vi "Periodic Tasks.vi"(8 "error in":errorcluster) -> ()   [LabVIEW 2019]
doc: "This VI runs in parallel to other tasks. It can contain as many user-defined periodic loops as you need. These can carry out PID or other sorts of timed response."
uses:
  <vilib>/Rock Robotics/WPI/Utilities/WPI_GetSetVariantRefNum.vi
  <vilib>/Rock Robotics/WPI/ThirdParty/Phoenix-LabVIEW/Motor Controller/Controls/CTRE_Phoenix_MotorControl_ControlMode.ctl
  <vilib>/Rock Robotics/WPI/ThirdParty/Phoenix-LabVIEW/Motor Controller/Controls/CTRE_Phoenix_MotorControl_RemoteFeedbackDevice.ctl
  <vilib>/Rock Robotics/WPI/ThirdParty/Phoenix-LabVIEW/Motor Controller/Controls/CTRE_Phoenix_MotorControl_RemoteSourceType.ctl
  <vilib>/Rock Robotics/WPI/ThirdParty/Phoenix-LabVIEW/Controls/CTRE_Phoenix_Params.ctl
panel:
  in  "Forward Limit Threshold":i32
  in  "Reverse Limit Threshold":i32
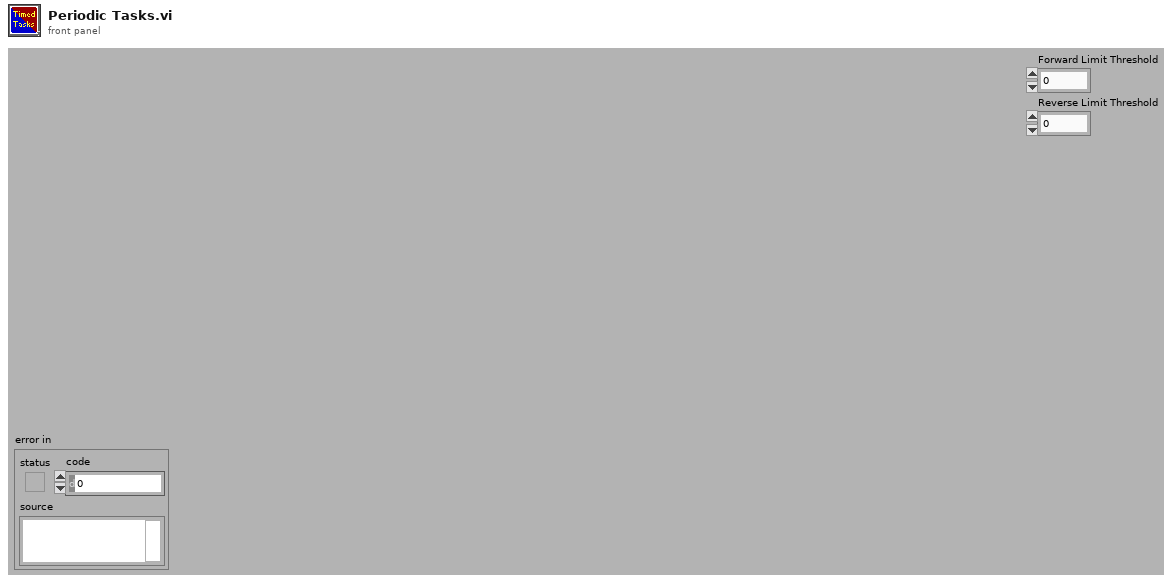
[diagram p1: front panel]
types:
  T1 = typedef "CTRE_PigeonIMU_DeviceRef.ctl" = cluster{"DeviceStatus":errorcluster, "Device Number":u8, "Type":T2, "Device ID":u32, "Handle":u64, "UsageFrame":u32, "Library Path":path}
  T2 = typedef "CTRE_PigeonIMU_ConnectionType.ctl" = u32
  T3 = typedef "CTRE_CANifier_DeviceRef.ctl" = cluster{"DeviceStatus":errorcluster, "Device Number":u8, "Handle":u64, "UsageFrame":u32, "Library Path":path}
  T4 = typedef "WPI_MotorControlDeviceRef.ctl" = cluster{"DeviceStatus":errorcluster, "Type":T5, "PWM":cluster{"PWM Channel":T6, "DeadBand":T7}, "CAN":cluster{"Device Number":u8, "SetOutput VI Ref":variant, "GetOutput VI Ref":variant, "Enable VI Ref":variant, "Disable VI Ref":variant, "Data":variant}, "Invert":bool, "DIO PWM":cluster{"PWM \"Enable\" Channel":T6, "DIOChannel":T8, "PWM Rate":dbl}}
  T5 = typedef "WPI_MotorControlType.ctl" = enum16{"PWM", "CAN", "DIO PWM"}
  T6 = typedef "FPGA_DIOPWMChannel.ctl" = enum8{"PWM 0", "PWM 1", "PWM 2", "PWM 3", "PWM 4", "PWM 5", "PWM 6", "PWM 7", "PWM 8", "PWM 9", "PWM MXP 0", "PWM MXP 1", "PWM MXP 2", "PWM MXP 3", "PWM MXP 4", "PWM MXP 5", "PWM MXP 6", "PWM MXP 7", "PWM MXP 8", "PWM MXP 9", "Invalid"}
  T7 = typedef "WPI_PWMDeadband.ctl" = cluster{"Name":string, "maxPositivePwm":i32, "minPositivePwm":i32, "centerPwm":i32, "maxNegativePwm":i32, "minNegativePwm":i32, "angularRange":u16}
  T8 = typedef "FPGA_DIOChannel.ctl" = enum8{"DIO 0", "DIO 1", "DIO 2", "DIO 3", "DIO 4", "DIO 5", "DIO 6", "DIO 7", "DIO 8", "DIO 9", "DIO MXP 0", "DIO MXP 1", "DIO MXP 2", "DIO MXP 3", "DIO MXP 4", "DIO MXP 5", "DIO MXP 6", "DIO MXP 7", "DIO MXP 8", "DIO MXP 9", "DIO MXP 10", "DIO MXP 11", "DIO MXP 12", "DIO MXP 13", "DIO MXP 14", "DIO MXP 15", "SPI Port CS1", "SPI Port CS2", "SPI Port CS3", "SPI Port MISO", "SPI Port MOSI", "Invalid"}
  T9 = typedef "WPI_JoystickDevRef.ctl" = cluster{"Device":T10}
  T10 = typedef "WPI_JoystickDeviceEnum.ctl" = enum16{"USB 0", "USB 1", "USB 2", "USB 3", "USB 4", "USB 5"}
  T11 = typedef "CTRE_Phoenix_MotorControl_RemoteSourceType.ctl" = enum16{"Off", "Talon SRX Selected Sensor", "Pigeon IMU Yaw", "Pigeon IMU Pitch", "Pigeon IMU Roll", "CANifier Quadrature", "CANifier PWM Input 0", "CANifier PWM Input 1", "CANifier PWM Input 2", "CANifier PWM Input 3", "Gadgeteer Pigeon Yaw", "Gadgeteer Pigeon Pitch", "Gadgeteer Pigeon Roll"}
  T12 = typedef "CTRE_Phoenix_MotorControl_ControlMode.ctl" = u16
  T13 = typedef "CTRE_Phoenix_MotorControl_RemoteFeedbackDevice.ctl" = i8
  T14 = typedef "CTRE_Phoenix_Params.ctl" = u16
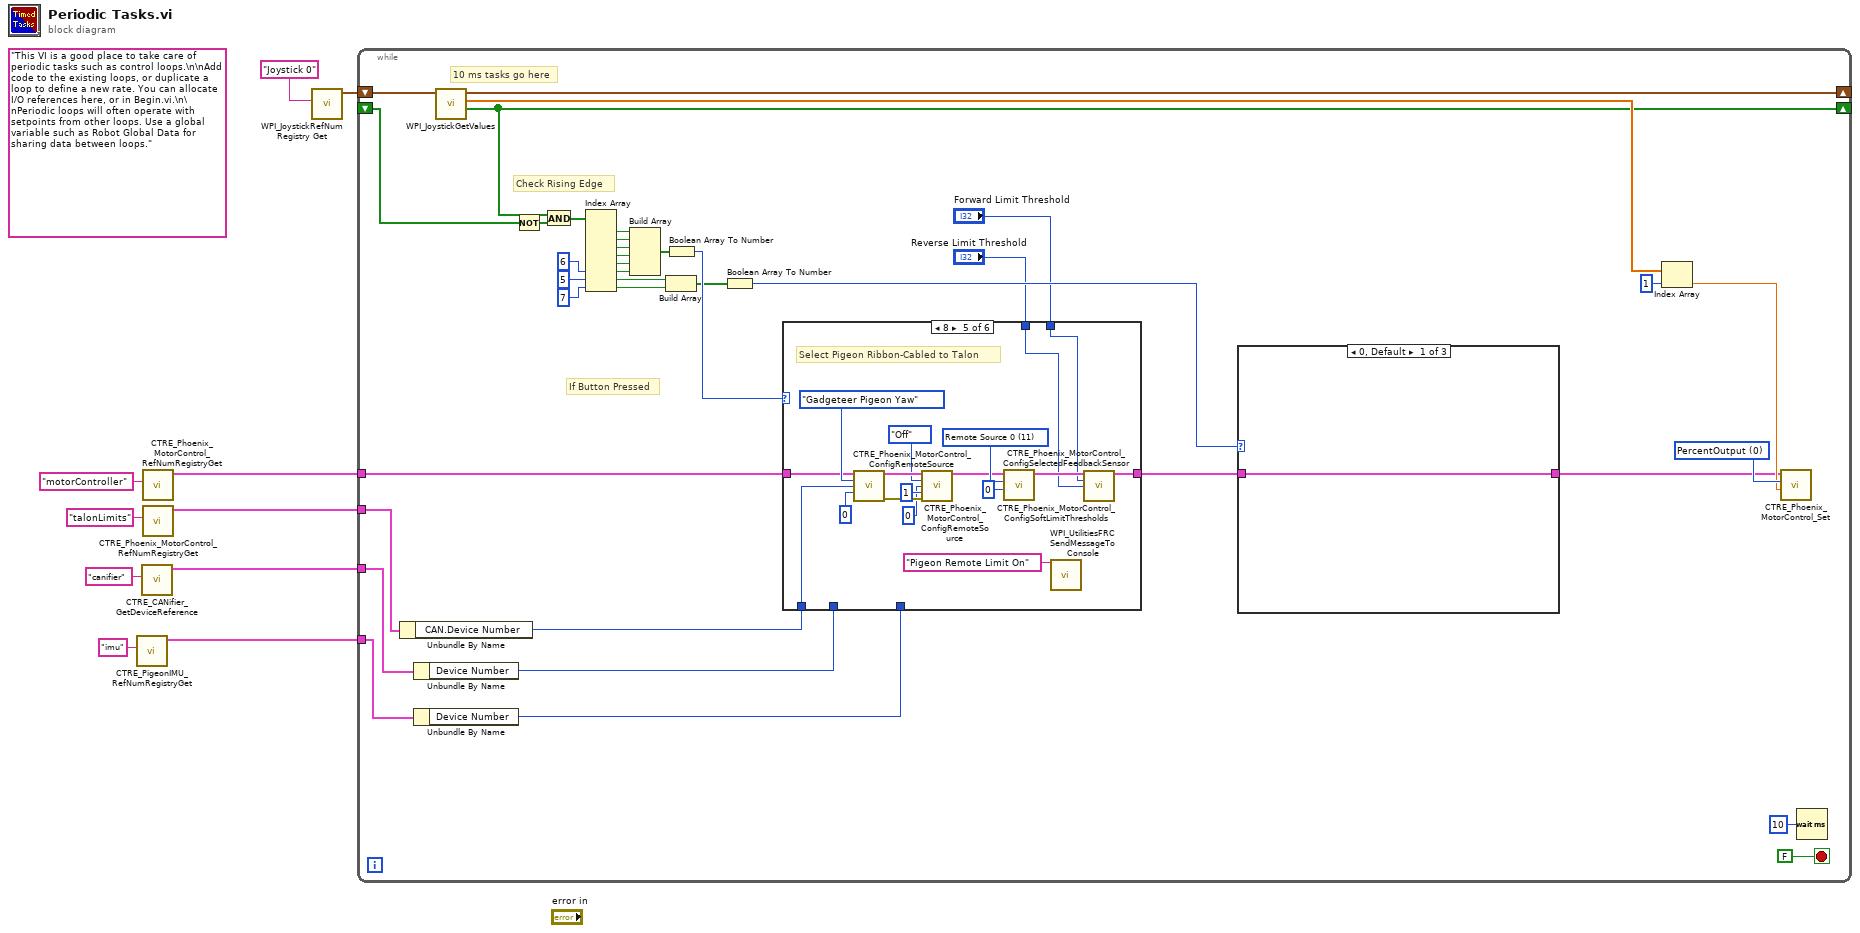
[diagram p0: block diagram]
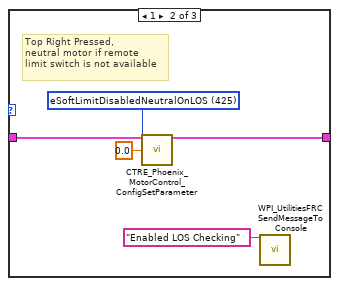
[diagram p2: hidden frame]
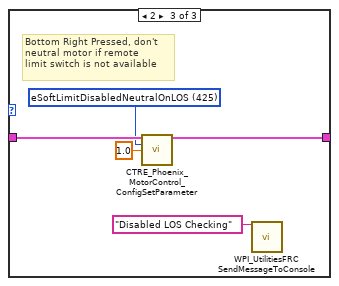
[diagram p3: hidden frame]
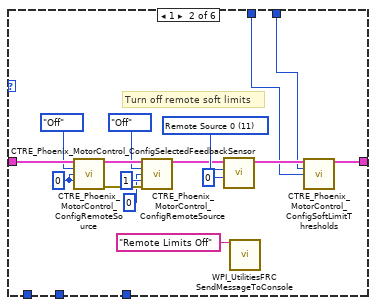
[diagram p5: hidden frame]
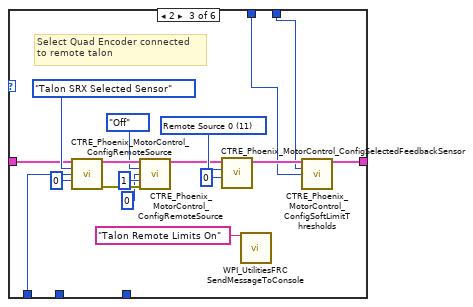
[diagram p6: hidden frame]
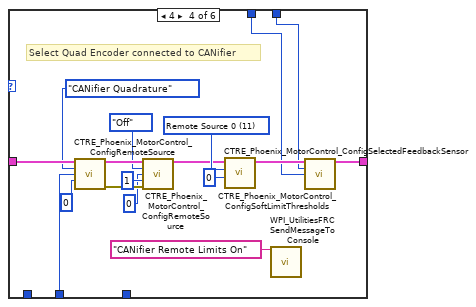
[diagram p7: hidden frame]
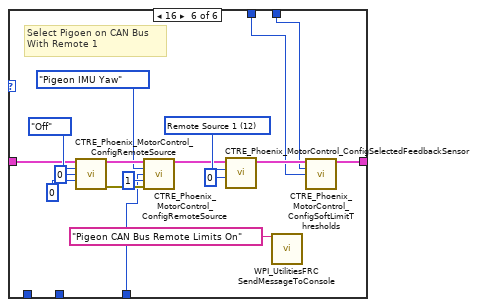
[diagram p8: hidden frame]
diagram:
  (unwired) "This VI is a good place to take care of periodic tasks such as control loops.\n\nAdd code to the existing loops, or duplicate a loop to define a new rate. You can allocate I/O references here, or in Begin.vi.\n\nPeriodic loops will often operate with setpoints from other loops. Use a global variable such as Robot Global Data for sharing data between loops."
  n1 = call <vilib>:"CTRE_PigeonIMU_RefNumRegistryGet.vi"("refnum name"="imu") -> ("PigeonIMUDevRef"=w1:T1)  [unwired: 9 in, 1 out]
  n2 = call <vilib>:"CTRE_CANifier_GetDeviceReference.vi"("refnum name"="canifier") -> ("CANifierDevRef"=w5:T3)  [unwired: 9 in, 1 out]
  n3 = call <vilib>:"CTRE_Phoenix_MotorControl_RefNumRegistryGet.vi"("refnum name"="motorController") -> ("PhoenixMotorControlDevRef"=w3:T4)  [unwired: 9 in, 1 out]
  n4 = call <vilib>:"CTRE_Phoenix_MotorControl_RefNumRegistryGet.vi"("refnum name"="talonLimits") -> ("PhoenixMotorControlDevRef"=w4:T4)  [unwired: 9 in, 1 out]
  n5 = call <vilib>:"WPI_JoystickRefNum Registry Get.vi"("refnum name"="Joystick 0") -> ("JoystickDevRef"=w9:T9)  [unwired: 1 in, 9 out]
  n6 = while {
    shift-right: [w44] -> _
    shift-left: w9 -> [w45]
    tunnel: w5 -> [w34]
    tunnel: w4 -> [w35]
    tunnel: w3 -> [w36]
    shift-right: [w39] -> _
    shift-left: _ -> [w40]
    tunnel: w1 -> [w12]
    stop <- FALSE stop-if-true
    w46 = T12 0 items=["PercentOutput"=0, "Position"=1, "Velocity"=2, "Current"=3, "Follower"=5, "MotionProfile"=6, "MotionMagic"=7, "MotionMagicArc"=8, "MotionProfileArc"=10, "Disabled"=15] ("Control Mode")
    # "If Button Pressed"
    # "Check Rising Edge"
    # "10 ms tasks go here"
    n7 = Unbundle By Name(w35) -> ("CAN.Device Number"=w27:u8)
    n8 = Unbundle By Name(w34) -> ("Device Number"=w26:u8)
    n9 = Unbundle By Name(w12) -> ("Device Number"=w11:u8)
    n10 = call <vilib>:"WPI_JoystickGetValues.vi"("JoystickDevRef"=w45) -> ("Buttons"=w39:bool[], "Axes"=w43:dbl[], "JoystickDevRef"=w44:T9)  [unwired: 6 in, 2 out]
    n11 = Not(x=w40) -> (.not. x?=w38:bool[])
    n12 = And(x=w39, y=w38) -> (x .and. y?=w37:bool[])
    n13 = Index Array(array=w37, index #6=6 ("index"), index #7=5 ("index"), index #8=7 ("index")) -> (element #1=w33:bool, element #2=w30:bool, element #3=w31:bool, element #4=w32:bool, element #5=w21:bool, element #6=w20:bool, element #7=w19:bool, element #8=w18:bool)  [unwired: 5 in]
    n14 = Build Array(w33, w30, w31, w32, w21, w20) -> (w29:bool[])
    n15 = Build Array(w19, w18) -> (w25:bool[])
    n16 = Boolean Array To Number(Boolean array=w29) -> (number=w28:u32)
    n17 = Boolean Array To Number(Boolean array=w25) -> (number=w23:u32)
    n18 = case shown="8" w28 {
      tunnel: w36 -> [w60 w75 w80 w100 w117 w134]
      tunnel: w27 -> [_ _ w84 _ w114 _]
      tunnel: w26 -> [_ _ _ w96 _ _]
      tunnel: [w60 w66 w79 w101 w118 w135] -> w22
      tunnel: "Reverse Limit Threshold" -> [_ w64 w82 w97 w116 w131]
      tunnel: "Forward Limit Threshold" -> [_ w65 w83 w98 w115 w132]
      tunnel: w11 -> [_ _ _ _ _ w133]
      frame 0, Default {
        # "Nothing pressed"
      }
      frame 1 {
        w62 = u32 0 ("Source Index (0/1)")
        w76 = T13 11 items=["None"=-1, "Sensor Sum (S0 + S1)"=9, "Sensor Difference (D0 - D1)"=10, "Remote Source 0"=11, "Remote Source 1"=12, "Software Emulated"=15] ("Feedback Device")
        # "Turn off remote soft limits"
        n19 = call <vilib>:"CTRE_Phoenix_MotorControl_ConfigRemoteSource.vi"("PhoenixMotorControlDevRef"=w75, "Remote Device Type"=CTRE_Phoenix_MotorControl_RemoteSourceType."Off", "Remote Device ID"=w62, "Source Index (0/1)"=w62) -> ("PhoenixMotorControlDevRef"=w72:T4, "error out"=w71:errorcluster)  [unwired: 10 in]
        n20 = call <vilib>:"CTRE_Phoenix_MotorControl_ConfigRemoteSource.vi"("PhoenixMotorControlDevRef"=w72, "Remote Device Type"=CTRE_Phoenix_MotorControl_RemoteSourceType."Off", "Remote Device ID"=u8 0, "Source Index (0/1)"=u32 1, "error in (no error)"=w71) -> ("PhoenixMotorControlDevRef"=w69:T4)  [unwired: 9 in, 1 out]
        n21 = call <vilib>:"CTRE_Phoenix_MotorControl_ConfigSelectedFeedbackSensor.vi"("pidLoopIdx"=0, "Feedback Device"=w76, "PhoenixMotorControlDevRef"=w69) -> ("PhoenixMotorControlDevRef"=w67:T4)  [unwired: 7 in, 1 out]
        n22 = call <vilib>:"WPI_UtilitiesFRC SendMessageToConsole.vi"("Message"="Remote Limits Off") -> ()  [unwired: 14 in, 1 out]
        n23 = call <vilib>:"CTRE_Phoenix_MotorControl_ConfigSoftLimitThresholds.vi"("PhoenixMotorControlDevRef"=w67, "Forward Soft Limit"=w65, "Reverse Soft Limit"=w64) -> ("PhoenixMotorControlDevRef"=w66:T4)  [unwired: 11 in, 1 out]
      }
      frame 2 {
        w93 = T13 11 items=["None"=-1, "Sensor Sum (S0 + S1)"=9, "Sensor Difference (D0 - D1)"=10, "Remote Source 0"=11, "Remote Source 1"=12, "Software Emulated"=15] ("Feedback Device")
        # "Select Quad Encoder connected\nto remote talon"
        n24 = call <vilib>:"CTRE_Phoenix_MotorControl_ConfigRemoteSource.vi"("PhoenixMotorControlDevRef"=w80, "Remote Device Type"=CTRE_Phoenix_MotorControl_RemoteSourceType."Talon SRX Selected Sensor", "Remote Device ID"=w84, "Source Index (0/1)"=u32 0) -> ("PhoenixMotorControlDevRef"=w90:T4, "error out"=w89:errorcluster)  [unwired: 10 in]
        n25 = call <vilib>:"CTRE_Phoenix_MotorControl_ConfigRemoteSource.vi"("PhoenixMotorControlDevRef"=w90, "Remote Device Type"=CTRE_Phoenix_MotorControl_RemoteSourceType."Off", "Remote Device ID"=u8 0, "Source Index (0/1)"=u32 1, "error in (no error)"=w89) -> ("PhoenixMotorControlDevRef"=w87:T4)  [unwired: 9 in, 1 out]
        n26 = call <vilib>:"CTRE_Phoenix_MotorControl_ConfigSelectedFeedbackSensor.vi"("pidLoopIdx"=0, "Feedback Device"=w93, "PhoenixMotorControlDevRef"=w87) -> ("PhoenixMotorControlDevRef"=w85:T4)  [unwired: 7 in, 1 out]
        n27 = call <vilib>:"WPI_UtilitiesFRC SendMessageToConsole.vi"("Message"="Talon Remote Limits On") -> ()  [unwired: 14 in, 1 out]
        n28 = call <vilib>:"CTRE_Phoenix_MotorControl_ConfigSoftLimitThresholds.vi"("PhoenixMotorControlDevRef"=w85, "Forward Soft Limit"=w83, "Reverse Soft Limit"=w82) -> ("PhoenixMotorControlDevRef"=w79:T4)  [unwired: 11 in, 1 out]
      }
      frame 4 {
        w110 = T13 11 items=["None"=-1, "Sensor Sum (S0 + S1)"=9, "Sensor Difference (D0 - D1)"=10, "Remote Source 0"=11, "Remote Source 1"=12, "Software Emulated"=15] ("Feedback Device")
        # "Select Quad Encoder connected to CANifier"
        n29 = call <vilib>:"CTRE_Phoenix_MotorControl_ConfigRemoteSource.vi"("PhoenixMotorControlDevRef"=w100, "Remote Device Type"=CTRE_Phoenix_MotorControl_RemoteSourceType."CANifier Quadrature", "Remote Device ID"=w96, "Source Index (0/1)"=u32 0) -> ("PhoenixMotorControlDevRef"=w108:T4, "error out"=w107:errorcluster)  [unwired: 10 in]
        n30 = call <vilib>:"CTRE_Phoenix_MotorControl_ConfigRemoteSource.vi"("PhoenixMotorControlDevRef"=w108, "Remote Device Type"=CTRE_Phoenix_MotorControl_RemoteSourceType."Off", "Remote Device ID"=u8 0, "Source Index (0/1)"=u32 1, "error in (no error)"=w107) -> ("PhoenixMotorControlDevRef"=w105:T4)  [unwired: 9 in, 1 out]
        n31 = call <vilib>:"CTRE_Phoenix_MotorControl_ConfigSelectedFeedbackSensor.vi"("pidLoopIdx"=0, "Feedback Device"=w110, "PhoenixMotorControlDevRef"=w105) -> ("PhoenixMotorControlDevRef"=w103:T4)  [unwired: 7 in, 1 out]
        n32 = call <vilib>:"WPI_UtilitiesFRC SendMessageToConsole.vi"("Message"="CANifier Remote Limits On") -> ()  [unwired: 14 in, 1 out]
        n33 = call <vilib>:"CTRE_Phoenix_MotorControl_ConfigSoftLimitThresholds.vi"("PhoenixMotorControlDevRef"=w103, "Forward Soft Limit"=w98, "Reverse Soft Limit"=w97) -> ("PhoenixMotorControlDevRef"=w101:T4)  [unwired: 11 in, 1 out]
      }
      frame 8 {
        w127 = T13 11 items=["None"=-1, "Sensor Sum (S0 + S1)"=9, "Sensor Difference (D0 - D1)"=10, "Remote Source 0"=11, "Remote Source 1"=12, "Software Emulated"=15] ("Feedback Device")
        # "Select Pigeon Ribbon-Cabled to Talon"
        n34 = call <vilib>:"CTRE_Phoenix_MotorControl_ConfigRemoteSource.vi"("PhoenixMotorControlDevRef"=w117, "Remote Device Type"=CTRE_Phoenix_MotorControl_RemoteSourceType."Gadgeteer Pigeon Yaw", "Remote Device ID"=w114, "Source Index (0/1)"=u32 0) -> ("PhoenixMotorControlDevRef"=w125:T4, "error out"=w124:errorcluster)  [unwired: 10 in]
        n35 = call <vilib>:"CTRE_Phoenix_MotorControl_ConfigRemoteSource.vi"("PhoenixMotorControlDevRef"=w125, "Remote Device Type"=CTRE_Phoenix_MotorControl_RemoteSourceType."Off", "Remote Device ID"=u8 0, "Source Index (0/1)"=u32 1, "error in (no error)"=w124) -> ("PhoenixMotorControlDevRef"=w122:T4)  [unwired: 9 in, 1 out]
        n36 = call <vilib>:"CTRE_Phoenix_MotorControl_ConfigSelectedFeedbackSensor.vi"("pidLoopIdx"=0, "Feedback Device"=w127, "PhoenixMotorControlDevRef"=w122) -> ("PhoenixMotorControlDevRef"=w120:T4)  [unwired: 7 in, 1 out]
        n37 = call <vilib>:"WPI_UtilitiesFRC SendMessageToConsole.vi"("Message"="Pigeon Remote Limit On") -> ()  [unwired: 14 in, 1 out]
        n38 = call <vilib>:"CTRE_Phoenix_MotorControl_ConfigSoftLimitThresholds.vi"("PhoenixMotorControlDevRef"=w120, "Forward Soft Limit"=w115, "Reverse Soft Limit"=w116) -> ("PhoenixMotorControlDevRef"=w118:T4)  [unwired: 11 in, 1 out]
      }
      frame 16 {
        w144 = T13 12 items=["None"=-1, "Sensor Sum (S0 + S1)"=9, "Sensor Difference (D0 - D1)"=10, "Remote Source 0"=11, "Remote Source 1"=12, "Software Emulated"=15] ("Feedback Device")
        # "Select Pigoen on CAN Bus\nWith Remote 1"
        n39 = call <vilib>:"CTRE_Phoenix_MotorControl_ConfigRemoteSource.vi"("PhoenixMotorControlDevRef"=w134, "Remote Device Type"=CTRE_Phoenix_MotorControl_RemoteSourceType."Off", "Remote Device ID"=u8 0, "Source Index (0/1)"=u32 0) -> ("PhoenixMotorControlDevRef"=w142:T4, "error out"=w141:errorcluster)  [unwired: 10 in]
        n40 = call <vilib>:"CTRE_Phoenix_MotorControl_ConfigRemoteSource.vi"("PhoenixMotorControlDevRef"=w142, "Remote Device Type"=CTRE_Phoenix_MotorControl_RemoteSourceType."Pigeon IMU Yaw", "Remote Device ID"=w133, "Source Index (0/1)"=u32 1, "error in (no error)"=w141) -> ("PhoenixMotorControlDevRef"=w139:T4)  [unwired: 9 in, 1 out]
        n41 = call <vilib>:"CTRE_Phoenix_MotorControl_ConfigSelectedFeedbackSensor.vi"("pidLoopIdx"=0, "Feedback Device"=w144, "PhoenixMotorControlDevRef"=w139) -> ("PhoenixMotorControlDevRef"=w137:T4)  [unwired: 7 in, 1 out]
        n42 = call <vilib>:"WPI_UtilitiesFRC SendMessageToConsole.vi"("Message"="Pigeon CAN Bus Remote Limits On") -> ()  [unwired: 14 in, 1 out]
        n43 = call <vilib>:"CTRE_Phoenix_MotorControl_ConfigSoftLimitThresholds.vi"("PhoenixMotorControlDevRef"=w137, "Forward Soft Limit"=w132, "Reverse Soft Limit"=w131) -> ("PhoenixMotorControlDevRef"=w135:T4)  [unwired: 11 in, 1 out]
      }
    }
    n44 = case shown="0, Default" w23 {
      tunnel: [w49 w52 w57] -> w24
      tunnel: w22 -> [w49 w54 w59]
      frame 0, Default {
      }
      frame 1 {
        w51 = T14 425 items=["eOnBoot_BrakeMode"=31, "eQuadFilterEn"=91, "eQuadIdxPolarity"=108, "eClearPositionOnIdx"=100, "eMotionProfileHasUnderrunErr"=119, "eMotionProfileTrajectoryPointDurationMs"=120, "eClearPosOnLimitF"=144, "eClearPosOnLimitR"=145, "eStatusFramePeriod"=300, "eOpenLoopRamp"=301, "eClosedLoopRamp"=302, "eNeutralDeadband"=303, "ePeakPosOutput"=305, "eNominalPosOutput"=306, "ePeakNegOutput"=307, "eNominalNegOutput"=308, "eProfileParamSlot_P"=310, "eProfileParamSlot_I"=311, "eProfileParamSlot_D"=312, "eProfileParamSlot_F"=313, "eProfileParamSlot_IZone"=314, "eProfileParamSlot_AllowableErr"=315, "eProfileParamSlot_MaxIAccum"=316, "eClearPositionOnLimitF"=320, "eClearPositionOnLimitR"=321, "eClearPositionOnQuadIdx"=322, "eSampleVelocityPeriod"=325, "eSampleVelocityWindow"=326, "eFeedbackSensorType"=330, "eSelectedSensorPosition"=331, "eFeedbackNotContinuous"=332, "eRemoteSensorSource"=333, "eRemoteSensorDeviceID"=334, "eSensorTerm"=335, "eRemoteSensorClosedLoopDisableNeutralOnLOS"=336, "eForwardSoftLimitThreshold"=340, "eReverseSoftLimitThreshold"=341, "eForwardSoftLimitEnable"=342, "eReverseSoftLimitEnable"=343, "eNominalBatteryVoltage"=350, "eBatterVoltageFilterSize"=351, "eContinuousCurrentLimitAmps"=360, "eContinuousCurrentLimitMs"=361, "ePeakCurrentLimitAmps"=362, "eClosedLoopIAccum"=370, "eCustomParam"=380, "eStickyFaults"=390, "eAnalogPosition"=400, "eQuadraturePosition"=401, "ePulseWidthPosition"=402, "eMotMag_Accel"=410, "eMotMag_VelCruise"=411, "eLimitSwitchSource"=421, "eLimitSwitchNormClosedAndDis"=422, "eLimitSwitchDisabledNeutralOnLOS"=423, "eLimitSwitchRemoteDevID"=424, "eSoftLimitDisabledNeutralOnLOS"=425] ("Parameter")
        # "Top Right Pressed,\nneutral motor if remote\nlimit switch is not available"
        n45 = call <vilib>:"CTRE_Phoenix_MotorControl_ConfigSetParameter.vi"("PhoenixMotorControlDevRef"=w54, "Parameter"=w51, "value"=0.0) -> ("PhoenixMotorControlDevRef"=w52:T4)  [unwired: 11 in, 1 out]
        n46 = call <vilib>:"WPI_UtilitiesFRC SendMessageToConsole.vi"("Message"="Enabled LOS Checking") -> ()  [unwired: 14 in, 1 out]
      }
      frame 2 {
        w56 = T14 425 items=["eOnBoot_BrakeMode"=31, "eQuadFilterEn"=91, "eQuadIdxPolarity"=108, "eClearPositionOnIdx"=100, "eMotionProfileHasUnderrunErr"=119, "eMotionProfileTrajectoryPointDurationMs"=120, "eClearPosOnLimitF"=144, "eClearPosOnLimitR"=145, "eStatusFramePeriod"=300, "eOpenLoopRamp"=301, "eClosedLoopRamp"=302, "eNeutralDeadband"=303, "ePeakPosOutput"=305, "eNominalPosOutput"=306, "ePeakNegOutput"=307, "eNominalNegOutput"=308, "eProfileParamSlot_P"=310, "eProfileParamSlot_I"=311, "eProfileParamSlot_D"=312, "eProfileParamSlot_F"=313, "eProfileParamSlot_IZone"=314, "eProfileParamSlot_AllowableErr"=315, "eProfileParamSlot_MaxIAccum"=316, "eClearPositionOnLimitF"=320, "eClearPositionOnLimitR"=321, "eClearPositionOnQuadIdx"=322, "eSampleVelocityPeriod"=325, "eSampleVelocityWindow"=326, "eFeedbackSensorType"=330, "eSelectedSensorPosition"=331, "eFeedbackNotContinuous"=332, "eRemoteSensorSource"=333, "eRemoteSensorDeviceID"=334, "eSensorTerm"=335, "eRemoteSensorClosedLoopDisableNeutralOnLOS"=336, "eForwardSoftLimitThreshold"=340, "eReverseSoftLimitThreshold"=341, "eForwardSoftLimitEnable"=342, "eReverseSoftLimitEnable"=343, "eNominalBatteryVoltage"=350, "eBatterVoltageFilterSize"=351, "eContinuousCurrentLimitAmps"=360, "eContinuousCurrentLimitMs"=361, "ePeakCurrentLimitAmps"=362, "eClosedLoopIAccum"=370, "eCustomParam"=380, "eStickyFaults"=390, "eAnalogPosition"=400, "eQuadraturePosition"=401, "ePulseWidthPosition"=402, "eMotMag_Accel"=410, "eMotMag_VelCruise"=411, "eLimitSwitchSource"=421, "eLimitSwitchNormClosedAndDis"=422, "eLimitSwitchDisabledNeutralOnLOS"=423, "eLimitSwitchRemoteDevID"=424, "eSoftLimitDisabledNeutralOnLOS"=425] ("Parameter")
        # "Bottom Right Pressed, don't\nneutral motor if remote\nlimit switch is not available"
        n47 = call <vilib>:"CTRE_Phoenix_MotorControl_ConfigSetParameter.vi"("PhoenixMotorControlDevRef"=w59, "Parameter"=w56, "value"=1.0) -> ("PhoenixMotorControlDevRef"=w57:T4)  [unwired: 11 in, 1 out]
        n48 = call <vilib>:"WPI_UtilitiesFRC SendMessageToConsole.vi"("Message"="Disabled LOS Checking") -> ()  [unwired: 14 in, 1 out]
      }
    }
    n49 = Index Array(array=w43, index=1) -> (element=w41:dbl)
    n50 = call <vilib>:"CTRE_Phoenix_MotorControl_Set.vi"("Output"=w41, "Control Mode"=w46, "PhoenixMotorControlDevRef"=w24) -> ()  [unwired: 7 in, 2 out]
    n51 = Wait (ms)(milliseconds to wait=u32 10) -> ()  [unwired: 1 out]
  }
